vi "ControlMotorDefinePostion.vi"(4 "位置":T1) -> (1 "位置消息输出":refnum<queue>)   [LabVIEW 2018]
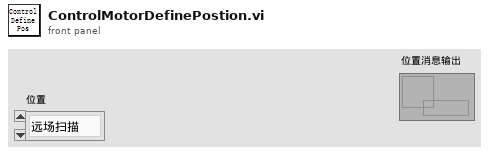
[diagram p1: front panel]
types:
  T1 = typedef "控制电机位置枚举器.ctl" = enum16{"远场扫描", "发散角扫描", "远场相机", "近场相机", "时间波形", "偏振", "能量", "功率", "光谱"}
  T2 = typedef "控制电机枚举器.ctl" = enum16{"Z", "Y", "X", "发散角", "俯仰", "旋转"}
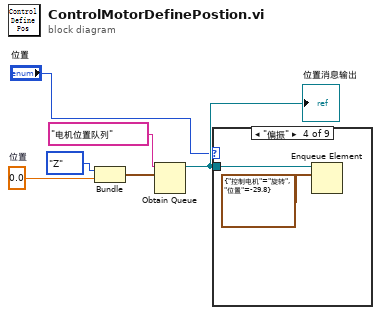
[diagram p0: block diagram]
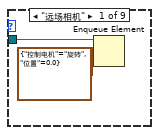
[diagram p2: hidden frame]
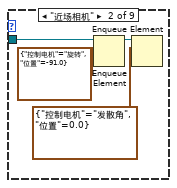
[diagram p3: hidden frame]
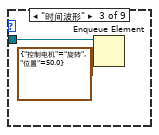
[diagram p4: hidden frame]
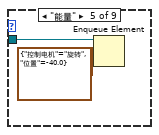
[diagram p5: hidden frame]
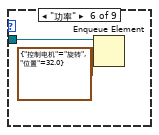
[diagram p6: hidden frame]
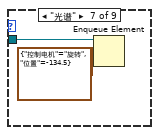
[diagram p7: hidden frame]
diagram:
  w5 = 0.0  # 位置
  n1 = Bundle("控制电机"=控制电机枚举器."Z", "位置"=w5) -> (w4:cluster{"控制电机":T2, "位置":dbl})  [unwired: 1 in]
  n2 = Obtain Queue(name (unnamed)="电机位置队列" ("名称（未命名）"), element data type=w4) -> (queue out=w3:refnum<queue>)  [unwired: 3 in, 2 out]
  "位置消息输出" <- w3
  n3 = case shown="\"偏振\"" "位置" {
    tunnel: w3 -> [w8 w12 w14 w16 w18 w20 w22 _ _]
    frame "远场相机" {
      n4 = Enqueue Element(queue=w8, element=cluster{"控制电机":T2, "位置":dbl} {"控制电机"=enum."旋转", "位置"=0.0} ("元素")) -> ()  [unwired: 2 in, 3 out]
    }
    frame "近场相机" {
      n5 = Enqueue Element(queue=w12, element=cluster{"控制电机":T2, "位置":dbl} {"控制电机"=enum."旋转", "位置"=-91.0} ("元素")) -> (queue out=w11:refnum<queue>)  [unwired: 2 in, 2 out]
      n6 = Enqueue Element(queue=w11, element=cluster{"控制电机":T2, "位置":dbl} {"控制电机"=enum."发散角", "位置"=0.0} ("元素")) -> ()  [unwired: 2 in, 3 out]
    }
    frame "时间波形" {
      n7 = Enqueue Element(queue=w14, element=cluster{"控制电机":T2, "位置":dbl} {"控制电机"=enum."旋转", "位置"=50.0} ("元素")) -> ()  [unwired: 2 in, 3 out]
    }
    frame "偏振" {
      n8 = Enqueue Element(queue=w16, element=cluster{"控制电机":T2, "位置":dbl} {"控制电机"=enum."旋转", "位置"=-29.8} ("元素")) -> ()  [unwired: 2 in, 3 out]
    }
    frame "能量" {
      n9 = Enqueue Element(queue=w18, element=cluster{"控制电机":T2, "位置":dbl} {"控制电机"=enum."旋转", "位置"=-40.0} ("元素")) -> ()  [unwired: 2 in, 3 out]
    }
    frame "功率" {
      n10 = Enqueue Element(queue=w20, element=cluster{"控制电机":T2, "位置":dbl} {"控制电机"=enum."旋转", "位置"=32.0} ("元素")) -> ()  [unwired: 2 in, 3 out]
    }
    frame "光谱" {
      n11 = Enqueue Element(queue=w22, element=cluster{"控制电机":T2, "位置":dbl} {"控制电机"=enum."旋转", "位置"=-134.5} ("元素")) -> ()  [unwired: 2 in, 3 out]
    }
    frame "远场扫描", Default {
    }
    frame "发散角扫描" {
    }
  }
